vi "Messaging Config.vi"(8 "error in (no error)":errorcluster, 11 "Cluster Config in":refnum<class "Cluster Config.lvclass">) -> (0 "error out":errorcluster, 2 "Messaging Config":T1, 3 "Cluster Config out":refnum<class "Cluster Config.lvclass">)   [LabVIEW 2020, in "VolatusConfig.lvlib" / "Cluster Config.lvclass"]
uses:
  Cluster Config.lvclass
  Cluster Config.lvclass/Cluster Config.ctl
  VolatusConfigElement/VolatusConfigElement.lvclass
  lv-cdm/CDM-Config/Config Element/Config Element.lvclass
  lv-vecto/VectoConfig/Endpoint.ctl
  lv-vecto/VectoConfig/VectoConfig.lvlib
  Messaging Config.ctl
  VolatusConfig.lvlib
  C:/dev/lv20CE/relink/lv-volatus/VolatusConfig/VolatusConfigElement/VolatusConfigElement.lvclass
  C:/dev/lv20CE/relink/lv-volatus/VolatusConfig/Cluster/Cluster Config.lvclass
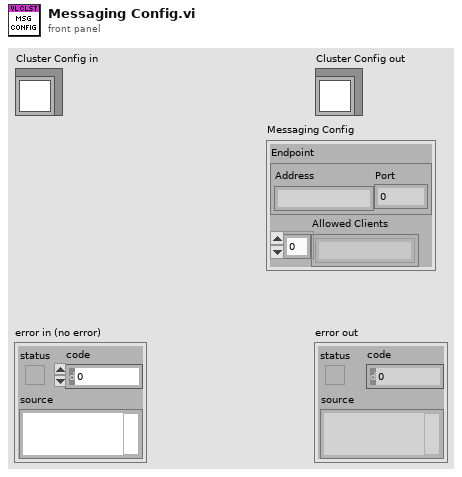
[diagram p1: front panel]
types:
  T1 = typedef "VolatusConfig.lvlib/Messaging Config.ctl" = cluster{"Endpoint":T2, "Allowed Clients":string[]}
  T2 = typedef "VectoConfig.lvlib/Endpoint.ctl" = cluster{"Address":string, "Port":u16}
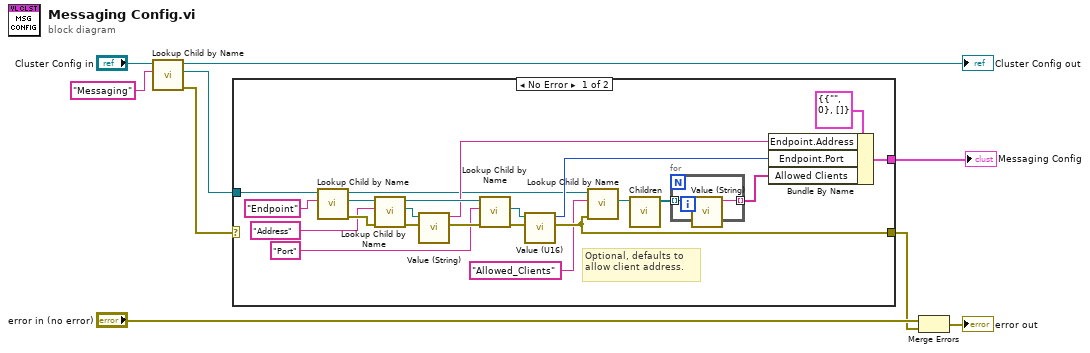
[diagram p0: block diagram]
diagram:
  n1 = call "Lookup Child by Name.vi"("Child Name"="Messaging", "VolatusConfigElement in"="Cluster Config in") -> ("error out"=w4:errorcluster, "Child"=w5:refnum<class "Config Element.lvclass">, "VolatusConfigElement out"=→"Cluster Config out":refnum<class "Cluster Config.lvclass">)  [unwired: 6 in, 1 out]
  n2 = case shown="No Error" w4 {
    tunnel: w5 -> [w19 _]
    tunnel: [w31 _] -> w1
    tunnel: [w15 _] -> w3
    frame No Error {
      # "Optional, defaults to allow client address."
      n3 = call "Lookup Child by Name.vi"("Name"="Endpoint", "Config Element in"=w19) -> ("error out"=w29:errorcluster, "Child"=w27:refnum<class "Config Element.lvclass">, "Config Element out"=w13:refnum<class "Config Element.lvclass">)  [unwired: 6 in, 1 out]
      n4 = call "Lookup Child by Name.vi"("error in (no error)"=w29, "Name"="Address", "Config Element in"=w27) -> ("error out"=w21:errorcluster, "Child"=w23:refnum<class "Config Element.lvclass">, "Config Element out"=w25:refnum<class "Config Element.lvclass">)  [unwired: 5 in, 1 out]
      n5 = call "Value (String).vi"("error in (no error)"=w21, "Config Element in"=w23) -> ("error out"=w30:errorcluster, "String Value"=w17:string)  [unwired: 8 in]
      n6 = call "Lookup Child by Name.vi"("error in (no error)"=w30, "Name"="Port", "Config Element in"=w25) -> ("error out"=w20:errorcluster, "Child"=w22:refnum<class "Config Element.lvclass">)  [unwired: 5 in, 2 out]
      n7 = call "Value (U16).vi"("error in (no error)"=w20, "Config Element in"=w22) -> ("error out"=w31:errorcluster, "U16 Value"=w16:u16)  [unwired: 8 in]
      n8 = call "Lookup Child by Name.vi"("error in (no error)"=w31, "Name"="Allowed_Clients", "Config Element in"=w13) -> ("Child"=w12:refnum<class "Config Element.lvclass">)  [unwired: 5 in, 3 out]
      n9 = call "Children.vi"("Config Element in"=w12) -> ("Elements"=w11:refnum<class "Config Element.lvclass">[])  [unwired: 9 in, 1 out]
      n10 = for {
        tunnel: w11 -> [w33] mode=indexing
        tunnel: [w32] -> w10 mode=indexing
        n11 = call "Value (String).vi"("Config Element in"=w33) -> ("String Value"=w32:string)  [unwired: 9 in, 1 out]
      }
      n12 = Bundle By Name(cluster=T1 {"Endpoint"={"Address"="", "Port"=0}, "Allowed Clients"=[]} ("Messaging Config"), "Endpoint.Address"=w17, "Endpoint.Port"=w16, "Allowed Clients"=w10) -> (w15:T1)
    }
    frame Error {
      # "No messaging config, is okay"
    }
  }
  "Messaging Config" <- w3
  n13 = Merge Errors("error in (no error)", w1) -> (→"error out":errorcluster)
